vi "EvalAndModifyLine.vi"(1 "path 2":T1[](array[typedef]) {"y" format="%.2f"; "x" format="%.2f"}, 4 "MaxLength":dbl) -> (14 "Ecxeeded":bool, 15 "path":T1[](array[typedef]) {"y" format="%.2f"; "x" format="%.2f"}, 16 "Point1_Can'tGoLeft":bool, 17 "Point1":T1 {"y" format="%.2f"; "x" format="%.2f"}, 18 "PointN-1":T1 {"y" format="%.2f"; "x" format="%.2f"}, 19 "PointN-1_Can'tGoLeft":bool)   [LabVIEW 2012, in "SegmentedLineEdge.lvclass"]
uses:
  <resource>/Framework/Providers/Open_GDS/UML/SegmentedLineEdge_class/SegmentedLineEdge.lvclass
  <resource>/Framework/Providers/Open_GDS/UML/General/Point/Point Point2D.ctl
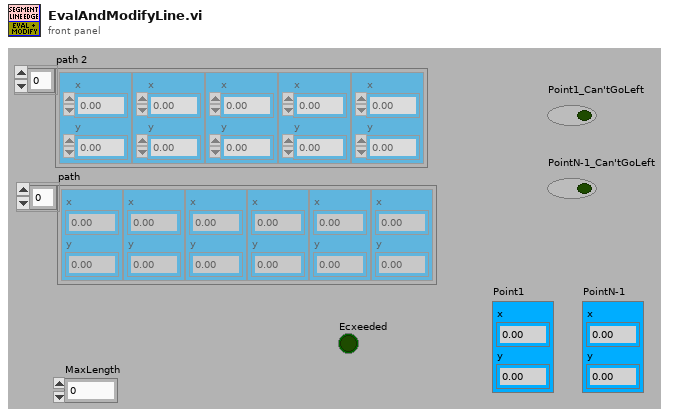
[diagram p1: front panel]
types:
  T1 = typedef "Point Point2D.ctl" = cluster{"x":dbl, "y":dbl}
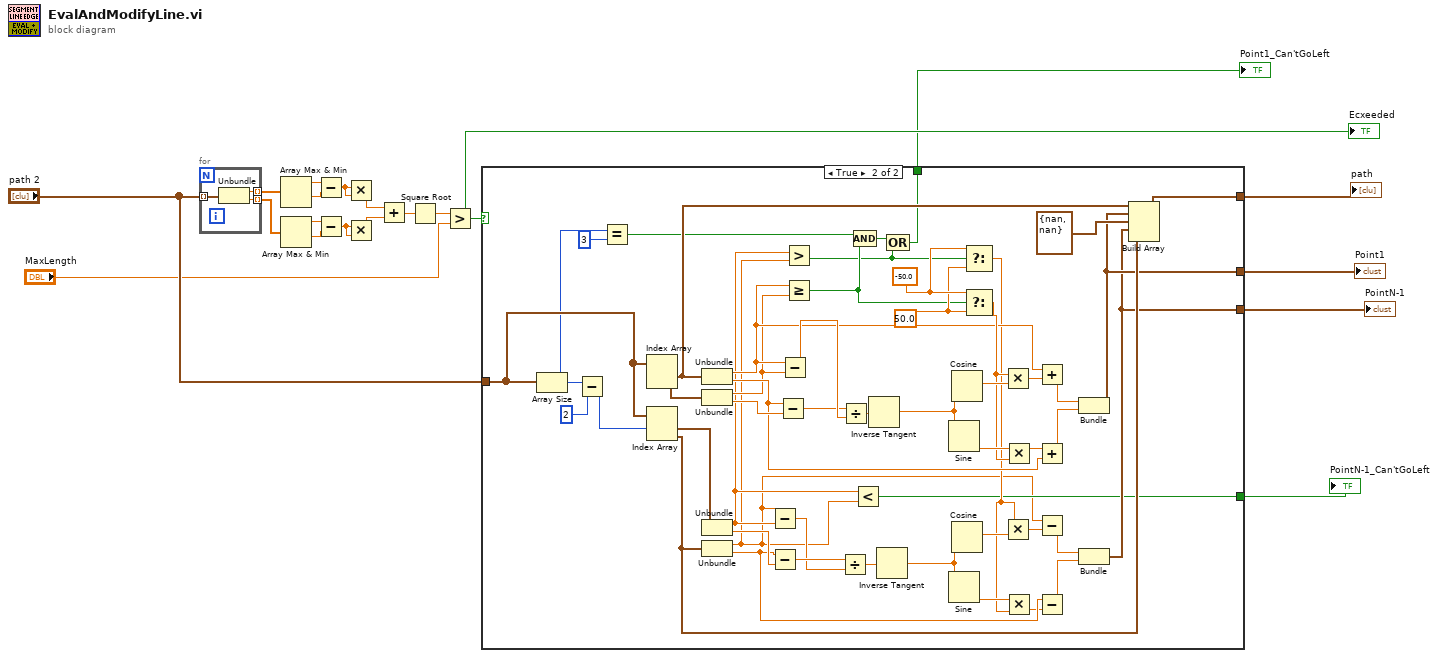
[diagram p0: block diagram]
diagram:
  n1 = for {
    tunnel: "path 2" -> [w23] mode=indexing
    tunnel: [w22] -> w7 mode=indexing
    tunnel: [w21] -> w8 mode=indexing
    n2 = Unbundle(w23) -> ("x"=w22:dbl, "y"=w21:dbl)
  }
  n3 = Array Max & Min(array=w7) -> (max value=w9:dbl, min value=w10:dbl)  [unwired: 2 out]
  n4 = Array Max & Min(array=w8) -> (max value=w11:dbl, min value=w12:dbl)  [unwired: 2 out]
  n5 = Subtract(x=w9, y=w10) -> (x-y=w6:dbl)
  n6 = Subtract(x=w11, y=w12) -> (x-y=w5:dbl)
  n7 = Multiply(x=w6, y=w6) -> (x*y=w4:dbl)
  n8 = Multiply(x=w5, y=w5) -> (x*y=w3:dbl)
  n9 = Add(x=w4, y=w3) -> (x+y=w2:dbl)
  n10 = Square Root(x=w2) -> (sqrt(x)=w1:dbl)
  n11 = Greater?(x=w1, y="MaxLength") -> (0:w17:bool)
  "Ecxeeded" <- w17
  n12 = case shown="True" w17 {
    tunnel: "path 2" -> [w24 w65]
    tunnel: [w24 w51] -> w19
    tunnel: [_ w43] -> w16
    tunnel: [_ w42] -> w15
    tunnel: [_ w31] -> w14
    tunnel: [_ w36] -> w13
    frame False {
    }
    frame True {
      w39 = 50.0 ("x")
      w40 = -50.0 ("x")
      n13 = Array Size(array=w65) -> (size(s)=w35:i32)
      n14 = Subtract(x=w35, y=2) -> (x-y=w67:i32)
      n15 = Equal?(x=w35, y=3) -> (x = y?=w33:bool)
      n16 = Index Array(array=w65) -> (element #1=w64:T1, element #2=w68:T1)  [unwired: 2 in]
      n17 = Index Array(array=w65, index #1=w67) -> (element #1=w53:T1, element #2=w52:T1)  [unwired: 1 in]
      n18 = Unbundle(w64) -> ("x"=w41:dbl, "y"=w47:dbl)
      n19 = Unbundle(w68) -> ("x"=w37:dbl, "y"=w48:dbl)
      n20 = Unbundle(w53) -> ("x"=w30:dbl, "y"=w56:dbl)
      n21 = Unbundle(w52) -> ("x"=w29:dbl, "y"=w50:dbl)
      n22 = Subtract(x=w29, y=w30) -> (x-y=w58:dbl)
      n23 = Subtract(x=w50, y=w56) -> (x-y=w60:dbl)
      n24 = Subtract(x=w47, y=w48) -> (x-y=w45:dbl)
      n25 = Subtract(x=w41, y=w37) -> (x-y=w46:dbl)
      n26 = Greater?(x=w30, y=w29) -> (0:w25:bool)
      n27 = Greater Or Equal?(x=w41, y=w37) -> (x >= y?=w26:bool)
      n28 = Divide(x=w60, y=w58) -> (x/y=w62:dbl)
      n29 = Divide(x=w45, y=w46) -> (x/y=w69:dbl)
      n30 = Less?(x=w30, y=w29) -> (x < y?=w36:bool)
      n31 = Compound Arithmetic op=AND(w33, w26) -> (w32:bool)
      n32 = Inverse Tangent(1:w69) -> (0:w28:dbl)
      n33 = Inverse Tangent(1:w62) -> (0:w27:dbl)
      n34 = Compound Arithmetic op=OR(w32, w25) -> (w31:bool)
      n35 = Sine(x=w28) -> (sin(x)=w70:dbl)
      n36 = Sine(x=w27) -> (sin(x)=w61:dbl)
      n37 = Cosine(x=w28) -> (cos(x)=w71:dbl)
      n38 = Cosine(x=w27) -> (cos(x)=w59:dbl)
      n39 = Select(t=w40, s=w25, f=w39) -> (s? t:f=w38:dbl)
      n40 = Select(t=w40, s=w26, f=w39) -> (s? t:f=w44:dbl)
      n41 = Multiply(x=w44, y=w71) -> (x*y=w72:dbl)
      n42 = Multiply(x=w38, y=w59) -> (x*y=w57:dbl)
      n43 = Multiply(x=w70, y=w44) -> (x*y=w73:dbl)
      n44 = Multiply(x=w61, y=w38) -> (x*y=w49:dbl)
      n45 = Add(x=w41, y=w72) -> (x+y=w74:dbl)
      n46 = Add(x=w73, y=w47) -> (x+y=w75:dbl)
      n47 = Subtract(x=w29, y=w57) -> (x-y=w55:dbl)
      n48 = Subtract(x=w50, y=w49) -> (x-y=w54:dbl)
      n49 = Bundle(w74, w75) -> (w43:cluster{dbl, dbl})  [unwired: 1 out]
      n50 = Bundle(w55, w54) -> (w42:cluster{dbl, dbl})  [unwired: 1 out]
      n51 = Build Array(w64, w43, T1 {"x"=nan, "y"=nan} ("element"), w42, w52) -> (w51:T1[])
    }
  }
  "path" <- w19
  "PointN-1" <- w15
  "Point1" <- w16
  "Point1_Can'tGoLeft" <- w14
  "PointN-1_Can'tGoLeft" <- w13
